vi "calculate_robot_position.vi"(2 "arc length angle":u16, 3 "Turning Radius (in)":fxp<+/-,22,12> format="%.14g") -> (0 "New Y Position":i16, 1 "New X Position":i16)   [LabVIEW 2009]
uses:
  <vilib>/Platform/TimedLoop/XDataNode/XDataNode.xnode
  <vilib>/Platform/TimedLoop/XDataNode/loadlvalarms.vi
  <vilib>/Platform/TimedLoop/XDataNode/timing_clust.ctl
  <vilib>/Platform/TimedLoop/XDataNode/nitl_modes.ctl
  <vilib>/Platform/TimedLoop/XDataNode/wakeup.ctl
  <vilib>/Platform/TimedLoop/XDataNode/XDNodeRunTimeDep.lvlib
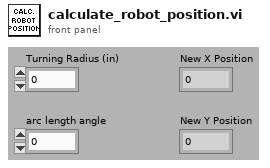
[diagram p1: front panel]
types:
  T1 = typedef "XDNodeRunTimeDep.lvlib/timing_clust.ctl" = cluster{"Expected End [f-1]":u64, "Actual End [f-1]":u64, "Finished Late? [f-1]":bool, "Expected End [i-1]":u64, "Actual End [i-1]":u64, "Finished Late? [i-1]":bool, "Expected Start [i]":u64, "Actual Start [i]":u64, "Expected Start [f]":u64, "Actual Start [f]":u64, "Source Name":string, "Structure Name":string, "Period":i64, "Deadline":i64, "Offset":i64, "Start":i64, "Priority":i32, "Timeout":i32, "Mode":T2, "Wakeup Reason":T3, "Error":errorcluster, "Source Type":string, "Secondary Source Type":string, "Global End Time":u64, "Global Start Time":u64, "Frame Duration":u64, "Iteration Duration":u64, "Assigned CPU":i32, "I/O Scan Engine Mode":u32}
  T2 = typedef "XDNodeRunTimeDep.lvlib/nitl_modes.ctl" = enum32{"No Change", "Process missed periods, maintain original phase", "Discard missed periods, maintain original phase", "Process missed periods, ignore original phase", "Discard missed periods, ignore original phase"}
  T3 = typedef "XDNodeRunTimeDep.lvlib/wakeup.ctl" = enum32{"Normal", "Aborted", "Asynchronous wakeup", "Timing source error", "Timed loop error", "Timeout"}
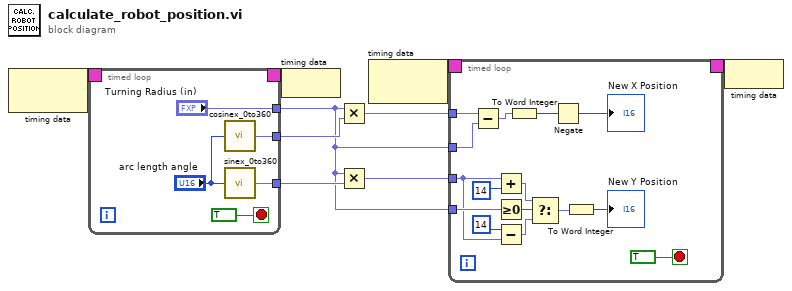
[diagram p0: block diagram]
diagram:
  n1 = node-c288() -> (w7:T1)  [unwired: 1 in]
  n2 = timed-loop {
    timing: w7 -> [_]
    timing-out: [_] -> w6
    tunnel: [w14] -> w9
    tunnel: [w13] -> w8
    tunnel: ["Turning Radius (in)"] -> w1
    stop <- TRUE stop-if-true
    n3 = call "cosinex_0to360.vi"("theta"="arc length angle") -> ("Numeric"=w13:fxp<+/-,16,1>)
    n4 = call "sinex_0to360.vi"("theta"="arc length angle") -> ("Numeric"=w14:fxp<+/-,16,1>)
  }
  n5 = node-c288(w6) -> ()
  n6 = Multiply(x=w1, y=w8) -> (x*y=w4:fxp<+/-,16,16>)
  n7 = Multiply(x=w1, y=w9) -> (x*y=w5:fxp<+/-,38,13>)
  n8 = node-c288() -> (w3:T1)  [unwired: 1 in]
  n9 = timed-loop {
    timing: w3 -> [_]
    timing-out: [_] -> w2
    tunnel: w1 -> [w31]
    tunnel: w5 -> [w21]
    tunnel: w4 -> [w18]
    tunnel: w1 -> [w25]
    stop <- TRUE stop-if-true
    n10 = Subtract(x=w18, y=w31) -> (x-y=w27:fxp<+/-,27,17>)
    n11 = Add(x=w21, y=i16 14) -> (x+y=w20:fxp<+/-,16,16>)
    n12 = Greater Or Equal To 0?(x=w25) -> (x >= 0?=w24:bool)
    n13 = Subtract(x=i16 14 ("y"), y=w21) -> (x-y=w19:fxp<+/-,42,17>)
    n14 = To Word Integer(number=w27) -> (16bit integer=w28:i16)
    n15 = Select(t=w20, s=w24, f=w19) -> (s? t:f=w23:fxp<+/-,42,17>)
    n16 = Negate(x=w28) -> (-x=→"New X Position":i16)
    n17 = To Word Integer(number=w23) -> (16bit integer=→"New Y Position":i16)
  }
  n18 = node-c288(w2) -> ()
